vi "ATF Storage-Datalog Redundant NS creater.vi"(9 "Data FIFO Ref":T1) -> ()   [LabVIEW 2022 SP3]
uses:
  RT Controls/ATF Storage-Data FIFO.ctl
  RT Controls/ATF Storage-DiplayPC comm ctrl.ctl
  <vilib>/dex/Stream Element Allocation Mode.ctl
  ATF Storage-RT_Global_R.vi
  <resource>/objmgr/ni.dex.rc
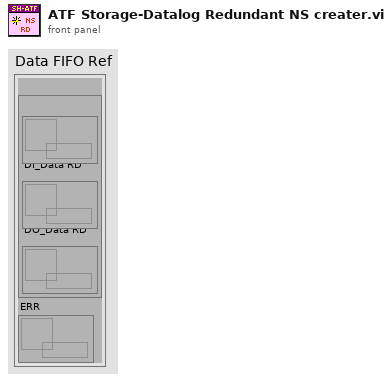
[diagram p1: front panel]
types:
  T1 = typedef "ATF Storage-Data FIFO.ctl" = cluster{"RD":cluster{"AI_V_Data RD":refnum<queue>, "DI_Data RD":refnum<queue>, "DO_Data RD":refnum<queue>}, "ERR":refnum<queue>}
  T2 = typedef "ATF Storage-DiplayPC comm ctrl.ctl" = enum16{"Initialize", "Listen for UI Writer", "Send RT Data"}
  T3 = typedef "Stream Element Allocation Mode.ctl" = u32
  T4 = cluster{"Start DAQ":bool, "Stop DAQ":bool, "RT Stop":bool, "RT Exit":bool, "Start Seq":bool}
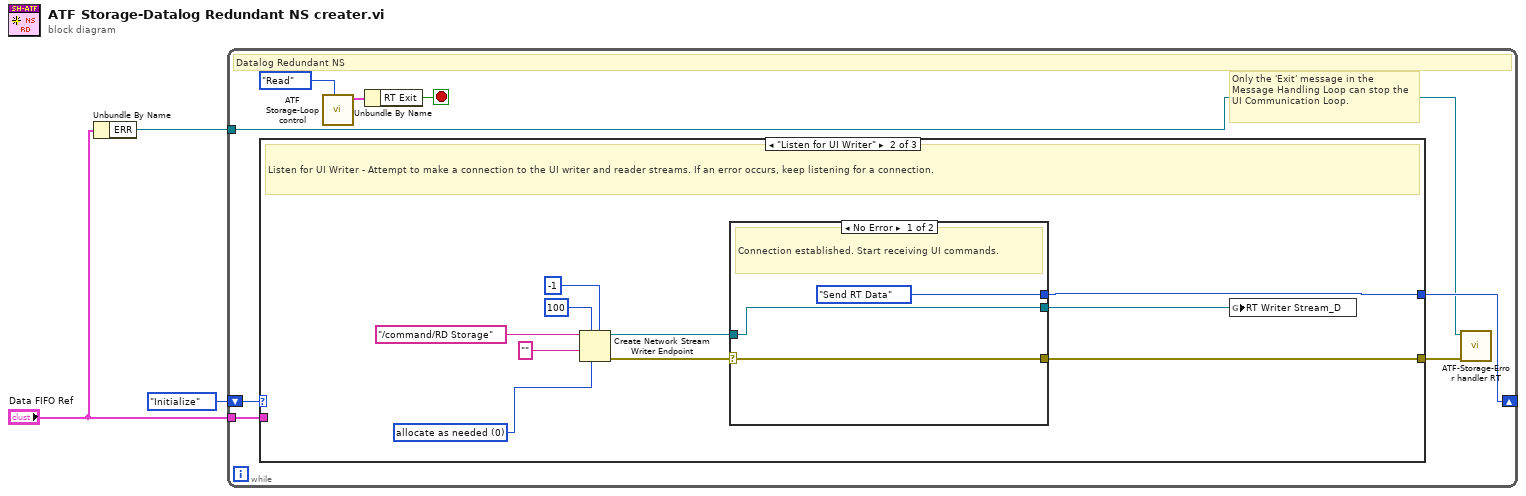
[diagram p0: block diagram]
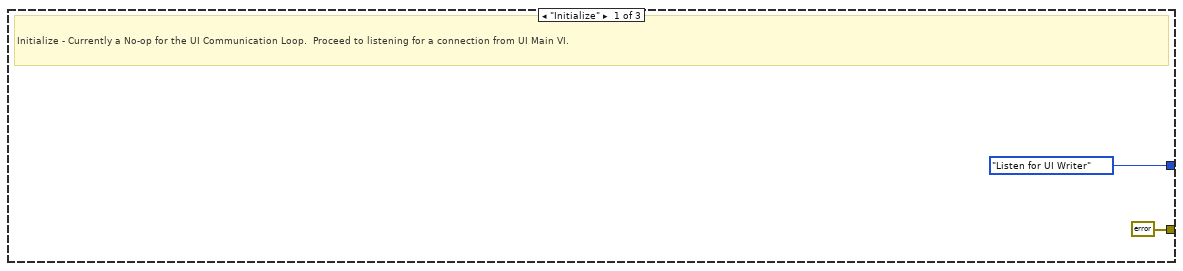
[diagram p2: hidden frame]
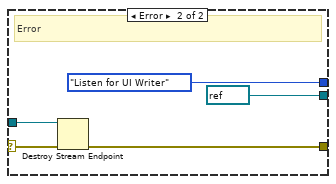
[diagram p3: hidden frame]
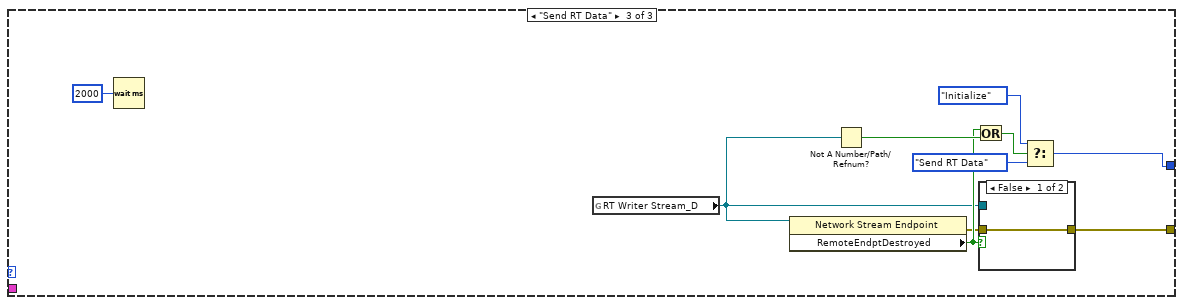
[diagram p4: hidden frame]
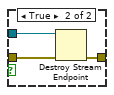
[diagram p5: hidden frame]
diagram:
  n1 = Unbundle By Name("Data FIFO Ref") -> ("ERR"=w2:refnum<queue>)
  n2 = while {
    shift-right: [w11] -> _
    shift-left: ATF_Storage-DiplayPC_comm_ctrl."Initialize" -> [w10]
    tunnel: "Data FIFO Ref" -> [w9]
    tunnel: w2 -> [w5]
    stop <- w6 stop-if-true
    # "Only the 'Exit' message in the  Message Handling Loop can stop the UI Communication Loop."
    # "Datalog Redundant NS"
    n3 = case shown="\"Listen for UI Writer\"" w10 {
      tunnel: [errorcluster {"status"=FALSE, "code"=0, "source"=""} ("error IO") w16 w32] -> w4
      tunnel: [ATF_Storage-DiplayPC_comm_ctrl."Listen for UI Writer" w21 w39] -> w11
      tunnel: w9 -> [_ _ _]
      frame "Initialize" {
        # "Initialize - Currently a No-op for the UI Communication Loop.  Proceed to listening for a connection from UI Main VI."
      }
      frame "Listen for UI Writer" {
        w14 = T3 0 items=["allocate as needed", "pre-allocate"] ("element allocation mode")
        # "Listen for UI Writer - Attempt to make a connection to the UI writer and reader streams. If an error occurs, keep listening for a connection."
        n4 = Create Network Stream Writer Endpoint(5:-1 ("timeout in ms (-1)"), 6:w14, 7:100 ("writer buffer size"), 9:"" ("reader url"), 11:"/command/RD Storage" ("reader url")) -> (0:w22:errorcluster, 3:w23:refnum<k21>)  [unwired: 2 in]
        n5 = case shown="No Error" w22 {
          selector: w22 -> [w24 w29]
          tunnel: w23 -> [w25 w31]
          tunnel: [ATF_Storage-DiplayPC_comm_ctrl."Send RT Data" ATF_Storage-DiplayPC_comm_ctrl."Listen for UI Writer"] -> w21
          tunnel: [w25 refnum<k21> refnum ("reader url")] -> w17
          tunnel: [w24 w27] -> w16
          frame No Error {
            # "Connection established. Start receiving UI commands."
          }
          frame Error {
            # "Error"
            n6 = Destroy Stream Endpoint(8:w29, 11:w31) -> (0:w27:errorcluster)
          }
        }
        n7 = global write "ATF Storage-RT_Global_R.vi" "RT Writer Stream_D"(w17) -> ()
      }
      frame "Send RT Data" {
        n8 = Wait (ms)(milliseconds to wait=u32 2000) -> ()  [unwired: 1 out]
        n9 = global read "ATF Storage-RT_Global_R.vi" "RT Writer Stream_D"() -> (w34:refnum<k21>)
        n10 = property class="Network Stream Endpoint"(reference=w34) -> (error out=w33:errorcluster, "RemoteEndptDestroyed"=w35:bool)  [unwired: 1 in, 1 out]
        n11 = Not A Number/Path/Refnum?(number/path/refnum=w34) -> (NaN/Path/Refnum?=w38:bool)
        n12 = Or(x=w35, y=w38) -> (x .or. y?=w37:bool)
        n13 = case shown="False" w35 {
          tunnel: w34 -> [_ w45]
          tunnel: w33 -> [w42 w44]
          tunnel: [w42 w43] -> w32
          frame False {
          }
          frame True {
            n14 = Destroy Stream Endpoint(8:w44, 11:w45) -> (0:w43:errorcluster)
          }
        }
        n15 = Select(t=ATF_Storage-DiplayPC_comm_ctrl."Initialize", s=w37, f=ATF_Storage-DiplayPC_comm_ctrl."Send RT Data") -> (s? t:f=w39:T2)
      }
    }
    n16 = call "ATF Storage-Loop control.vi"("Action"=enum16{"Init", "Write", "Read"}."Read") -> ("Loop Control out"=w8:T4)  [unwired: 9 in, 1 out]
    n17 = Unbundle By Name(w8) -> ("RT Exit"=w6:bool)
    n18 = call "ATF-Storage-Error handler RT.vi"("error in"=w4, "Message Queue"=w5) -> ()  [unwired: 8 in, 2 out]
  }
